vi "From JSON.vi"(7 "LVClass Serializer":refnum<class "JSONtext LVClass Serializer.lvclass">, 8 "error in (no error)":errorcluster, 10 "<JSON>":string, 11 "Serializable Account in":refnum<class "Serializable Account.lvclass">) -> (0 "error out":errorcluster, 3 "Serializable Account out":refnum<class "Serializable Account.lvclass">)   [LabVIEW 2017, in "Serializable Account.lvclass"]
doc: "Reads data from a JSON string."
uses:
  Serializable Account.lvclass
  <vilib>/JDP Science/JSONtext/LVClass Serializer/JSONtext LVClass Serializer.lvclass
  Serializable Account.lvclass/Serializable Account.ctl
  <vilib>/JDP Science/JSONtext/JSONtext.lvlib
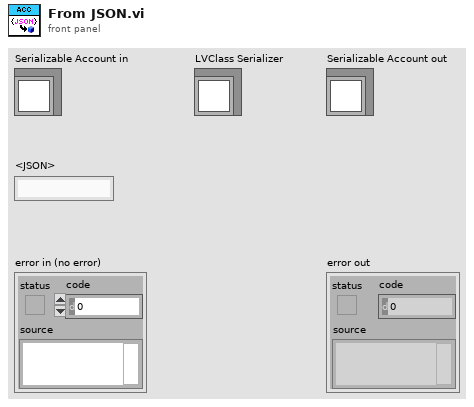
[diagram p1: front panel]
types:
  T1 = cluster{"MD5 message-digest":string, "Email":string, "Active":bool, "CreatedDate":timestamp, "Roles":string[]}
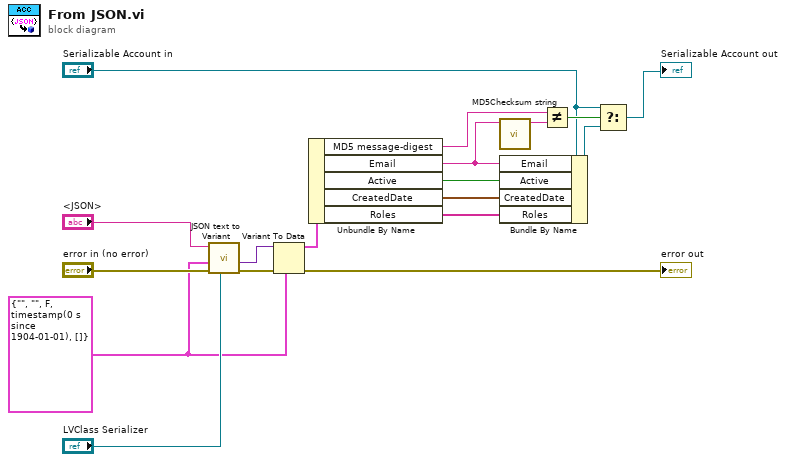
[diagram p0: block diagram]
diagram:
  w12 = T1 {"MD5 message-digest"="", "Email"="", "Active"=FALSE, "CreatedDate"=timestamp(0 s since 1904-01-01), "Roles"=[]} ("cluster")
  n1 = call <vilib>:"JSON text to Variant.vi"("LVClass Serializer"="LVClass Serializer", "error in (no error)"="error in (no error)", "Data Type"=w12, "JSON"="<JSON>") -> ("error out"=w16:errorcluster, "Variant out"=w13:variant)  [unwired: 6 in]
  n2 = Variant To Data(error in=w16, type=w12, Variant=w13) -> (data=w11:T1, error out=→"error out":errorcluster)
  n3 = Unbundle By Name(w11) -> ("MD5 message-digest"=w5:string, "Email"=w7:string, "Active"=w10:bool, "CreatedDate"=w9:timestamp, "Roles"=w8:string[])
  n4 = call <vilib>:"MD5Checksum string.vi"("Message String"=w7) -> ("MD5 message-digest"=w6:string)  [unwired: 10 in]
  n5 = Bundle By Name(cluster="Serializable Account in", "Email"=w7, "Active"=w10, "CreatedDate"=w9, "Roles"=w8) -> (w2:refnum<class "Serializable Account.lvclass">)
  n6 = Not Equal?(x=w5, y=w6) -> (x != y?=w4:bool)
  n7 = Select(t="Serializable Account in", s=w4, f=w2) -> (s? t:f=→"Serializable Account out":refnum<class "Serializable Account.lvclass">)
